vi "Variant to Datatype.vi"(4 "Variant":variant) -> (0 "Value":string, 1 "Name":string, 2 "Datatype":T1)   [LabVIEW 2019]
uses:
  Datatype.ctl
  <userlib>/_OpenG.lib/lvdata/lvdata.llb/Type Descriptor Enumeration__ogtk.ctl
  <vilib>/Utility/Data Type/NI_Data Type.lvlib
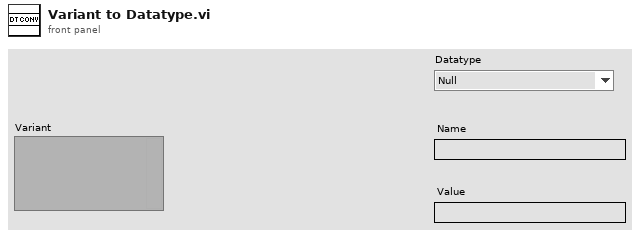
[diagram p1: front panel]
types:
  T1 = typedef "Datatype.ctl" = enum16{"Null", "Numeric", "String", "Bool", "Numeric 1D", "String 1D", "Bool 1D", "Numeric 2D", "String 2D", "Bool 2D", "Variant"}
  T2 = typedef "Type Descriptor Enumeration__ogtk.ctl" = enum8{"<Null>", "I8", "I16", "I32", "I64", "U8", "U16", "U32", "U64", "SGL", "DBL", "EXT", "CSG", "CDB", "CXT", "0x0F", "0x10", "0x11", "0x12", "0x13", "0x14", "Enum U8", "Enum U16", "Enum U32", "Enum U64", "SGL PQ", "DBL PQ", "EXT PQ", "CSG PQ", "CDB PQ", "CXT PQ", "0x1F", "0x20", "Boolean", "0x22", "0x23", "0x24", "0x25", "0x26", "0x27", "0x28", "0x29", "0x2A", "0x2B", "0x2C", "0x2D", "0x2E", "0x2F", "String", "0x31", "Path", "Pict", "0x34", "0x35", "0x36", "DAQ", "0x38", "0x39", "0x3A", "0x3B", "0x3C", "0x3D", "0x3E", "0x3F", "Array", "0x41", "0x42", "0x43", "0x44", "0x45", "0x46", "0x47", "0x48", "0x49", "0x4A", "0x4B", "0x4C", "0x4D", "0x4E", "0x4F", "Cluster", "0x51", "0x52", "Variant", "Waveform", "0x55", "0x56", "0x57", "0x58", "0x59", "0x5A", "0x5B", "0x5C", "0x5D", "0x5E", "Fixed Point", "0x60", "0x61", "0x62", "0x63", "0x64", "0x65", "0x66", "0x67", "0x68", "0x69", "0x6A", "0x6B", "0x6C", "0x6D", "0x6E", "0x6F", "Refnum", "0x71", "0x72", "Set Collection", "Map Collection"}
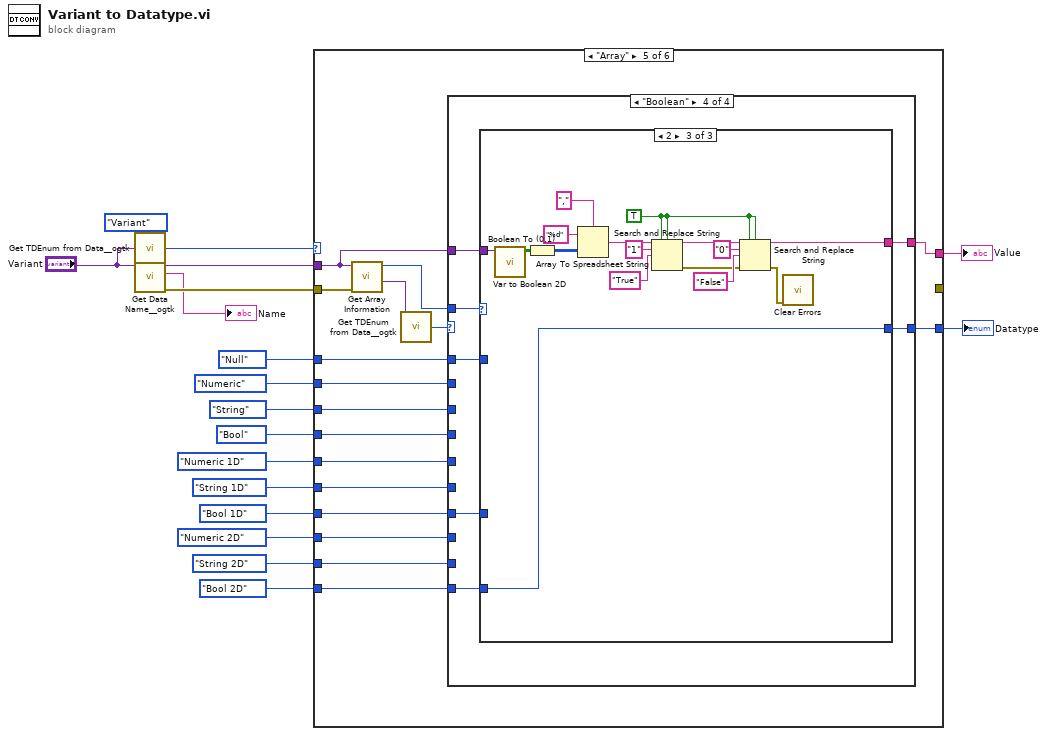
[diagram p0: block diagram]
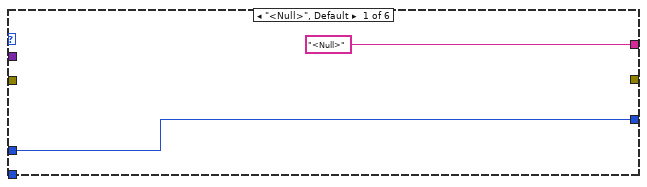
[diagram p2: hidden frame]
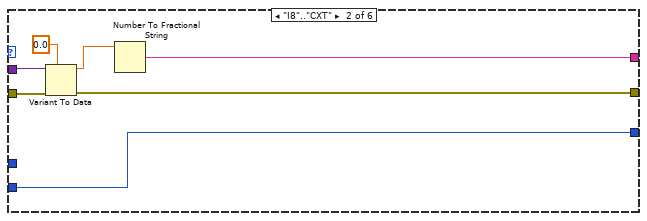
[diagram p3: hidden frame]
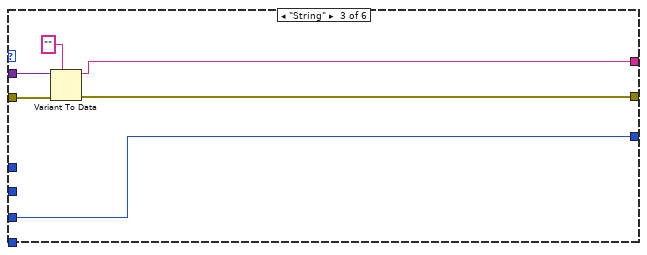
[diagram p4: hidden frame]
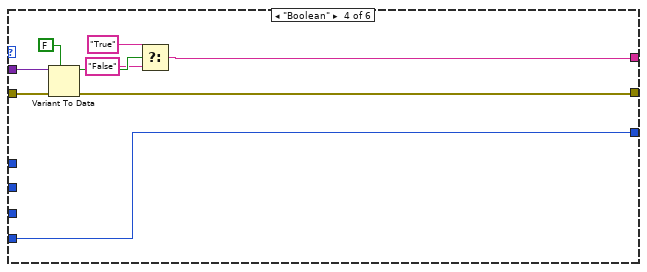
[diagram p5: hidden frame]
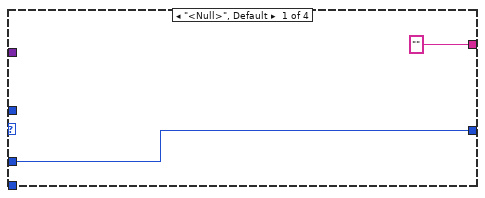
[diagram p6: hidden frame]
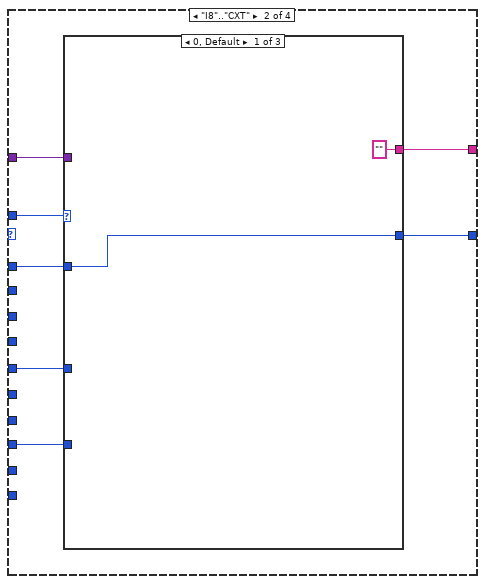
[diagram p7: hidden frame]
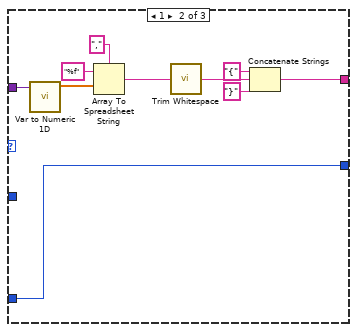
[diagram p8: hidden frame]
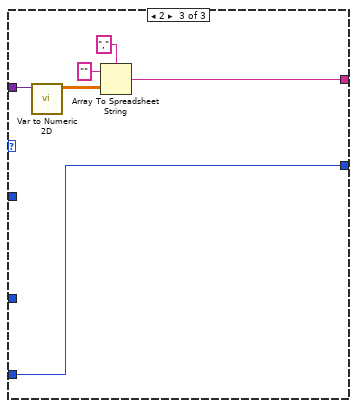
[diagram p9: hidden frame]
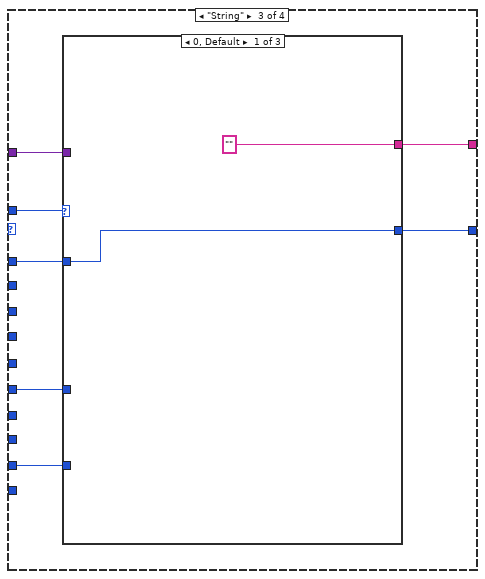
[diagram p10: hidden frame]
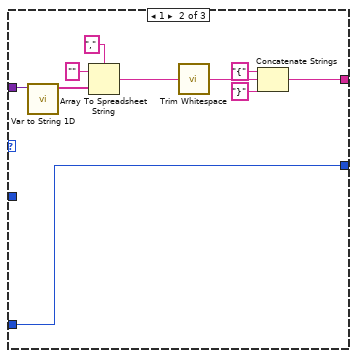
[diagram p11: hidden frame]
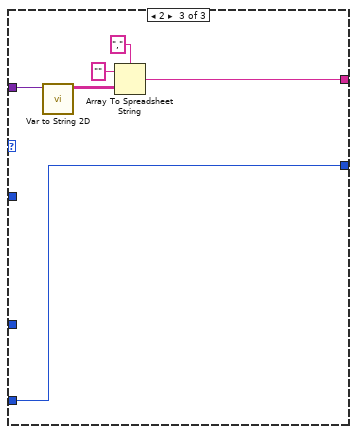
[diagram p12: hidden frame]
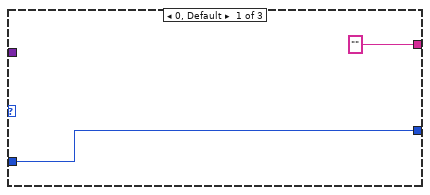
[diagram p13: hidden frame]
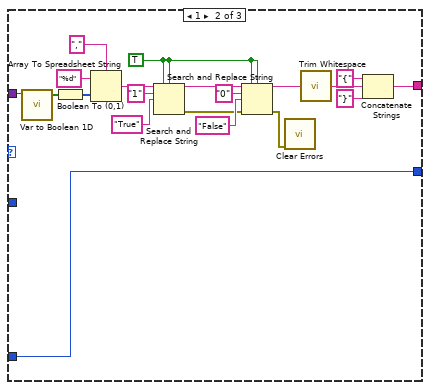
[diagram p14: hidden frame]
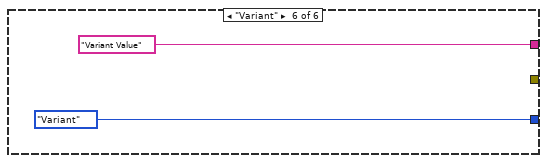
[diagram p15: hidden frame]
diagram:
  (unwired) Type_Descriptor_Enumeration__ogtk."Variant" ("Type Descriptor Enumeration")
  n1 = call <userlib>:"Get TDEnum from Data__ogtk.vi"("Data"="Variant") -> ("Type Descriptor Enumeration"=w11:T2)  [unwired: 4 in]
  n2 = call <userlib>:"Get Data Name__ogtk.vi"("Data"="Variant") -> ("error out"=w10:errorcluster, "Data Name"=→"Name":string, "Data dup"=w8:variant)  [unwired: 8 in]
  n3 = case shown="\"Array\"" w11 {
    tunnel: [w19 w26 w32 w41 w55 Datatype."Variant" ("Datatype")] -> w17
    tunnel: Datatype."Null" ("Datatype") -> [w19 _ _ _ w54 _]
    tunnel: Datatype."Numeric" ("Datatype") -> [_ w26 _ _ w53 _]
    tunnel: Datatype."String" ("Datatype") -> [_ _ w32 _ w52 _]
    tunnel: Datatype."Bool" ("Datatype") -> [_ _ _ w41 w51 _]
    tunnel: w10 -> [_ w24 w29 w38 w58 _]
    tunnel: w8 -> [_ w25 w30 w39 w43 _]
    tunnel: Datatype."Numeric 1D" ("Datatype") -> [_ _ _ _ w50 _]
    tunnel: Datatype."String 1D" ("Datatype") -> [_ _ _ _ w49 _]
    tunnel: Datatype."Bool 1D" ("Datatype") -> [_ _ _ _ w48 _]
    tunnel: Datatype."Numeric 2D" ("Datatype") -> [_ _ _ _ w47 _]
    tunnel: Datatype."String 2D" ("Datatype") -> [_ _ _ _ w46 _]
    tunnel: Datatype."Bool 2D" ("Datatype") -> [_ _ _ _ w45 _]
    tunnel: ["<Null>" w21 w28 w35 w42 "Variant Value"] -> w1
    tunnel: [_ w20 w27 w37 _ _] -> _
    frame "<Null>", Default {
    }
    frame "I8".."CXT" {
      n4 = Variant To Data(error in=w24, type=0.0, Variant=w25) -> (data=w22:dbl, error out=w20:errorcluster)
      n5 = Number To Fractional String(number=w22) -> (F-format string=w21:string)  [unwired: 3 in]
    }
    frame "String" {
      n6 = Variant To Data(error in=w29, type="", Variant=w30) -> (data=w28:string, error out=w27:errorcluster)
    }
    frame "Boolean" {
      n7 = Variant To Data(error in=w38, type=FALSE, Variant=w39) -> (data=w36:bool, error out=w37:errorcluster)
      n8 = Select(t="True", s=w36, f="False") -> (s? t:f=w35:string)
    }
    frame "Array" {
      n9 = call <vilib>:"Get Array Information.vi"("error in (no error)"=w58, "variant"=w43) -> ("array element data type"=w57:variant, "number of dimensions"=w44:i32)  [unwired: 6 in, 2 out]
      n10 = call <userlib>:"Get TDEnum from Data__ogtk.vi"("Data"=w57) -> ("Type Descriptor Enumeration"=w56:T2)  [unwired: 4 in]
      n11 = case shown="\"Boolean\"" w56 {
        tunnel: [w60 w61 w86 w116] -> w55
        tunnel: w54 -> [w60 w66 w92 w115]
        tunnel: w53 -> [_ _ _ _]
        tunnel: w52 -> [_ _ _ _]
        tunnel: w51 -> [_ _ _ _]
        tunnel: w50 -> [_ w65 _ _]
        tunnel: w49 -> [_ _ w90 _]
        tunnel: w48 -> [_ _ _ w114]
        tunnel: w47 -> [_ w64 _ _]
        tunnel: w46 -> [_ _ w89 _]
        tunnel: w45 -> [_ _ _ w113]
        tunnel: w44 -> [_ w67 w91 w117]
        tunnel: w43 -> [_ w63 w88 w112]
        tunnel: ["" ("spreadsheet string") w62 w87 w111] -> w42
        frame "<Null>", Default {
        }
        frame "I8".."CXT" {
          n12 = case shown="0, Default" w67 {
            tunnel: [w69 w79 w85] -> w61
            tunnel: w66 -> [w69 _ _]
            tunnel: w65 -> [_ w79 _]
            tunnel: w64 -> [_ _ w85]
            tunnel: w63 -> [_ w76 w81]
            tunnel: ["" w72 w82] -> w62
            frame 0, Default {
            }
            frame 1 {
              n13 = call "Var to Numeric 1D.vi"("Variant"=w76) -> ("Numeric Array"=w75:dbl[])  [unwired: 10 in]
              n14 = Array To Spreadsheet String(delimiter (Tab)=",", array=w75, 3:"%f" ("format string")) -> (spreadsheet string=w74:string)
              n15 = call <vilib>:"Trim Whitespace.vi"("string"=w74) -> ("trimmed string"=w73:string)  [unwired: 1 in]
              n16 = Concatenate Strings("{" ("string"), w73, "}" ("string")) -> (w72:string)
            }
            frame 2 {
              n17 = call "Var to Numeric 2D.vi"("Variant"=w81) -> ("Numeric Array"=w80:dbl[][])  [unwired: 10 in]
              n18 = Array To Spreadsheet String(delimiter (Tab)=",", array=w80, 3:"" ("format string")) -> (spreadsheet string=w82:string)
            }
          }
        }
        frame "String" {
          n19 = case shown="0, Default" w91 {
            tunnel: [w94 w104 w110] -> w86
            tunnel: w92 -> [w94 _ _]
            tunnel: w90 -> [_ w104 _]
            tunnel: w89 -> [_ _ w110]
            tunnel: w88 -> [_ w103 w107]
            tunnel: ["" ("spreadsheet string") w95 w105] -> w87
            frame 0, Default {
            }
            frame 1 {
              n20 = call "Var to String 1D.vi"("Variant"=w103) -> ("String 1D"=w102:string[])  [unwired: 10 in]
              n21 = Array To Spreadsheet String(delimiter (Tab)=",", array=w102, 3:"" ("format string")) -> (spreadsheet string=w96:string)
              n22 = call <vilib>:"Trim Whitespace.vi"("string"=w96) -> ("trimmed string"=w99:string)  [unwired: 1 in]
              n23 = Concatenate Strings("{" ("string"), w99, "}" ("string")) -> (w95:string)
            }
            frame 2 {
              n24 = call "Var to String 2D.vi"("Variant"=w107) -> ("String 2D"=w106:string[][])  [unwired: 10 in]
              n25 = Array To Spreadsheet String(delimiter (Tab)=",", array=w106, 3:"" ("format string")) -> (spreadsheet string=w105:string)
            }
          }
        }
        frame "Boolean" {
          n26 = case shown="2" w117 {
            tunnel: [w119 w139 w155] -> w116
            tunnel: w115 -> [w119 _ _]
            tunnel: w114 -> [_ w139 _]
            tunnel: w113 -> [_ _ w155]
            tunnel: w112 -> [_ w128 w141]
            tunnel: ["" w120 w142] -> w111
            frame 0, Default {
            }
            frame 1 {
              w129 = TRUE ("replace all? (F)")
              n27 = call "Var to Boolean 1D.vi"("Variant"=w128) -> ("Bool 1D"=w127:bool[])  [unwired: 10 in]
              n28 = Boolean To (0,1)(Boolean=w127) -> (0, 1=w138:i16[])
              n29 = Array To Spreadsheet String(delimiter (Tab)=",", array=w138, 3:"%d" ("format string")) -> (spreadsheet string=w135:string)
              n30 = Search and Replace String(replace all?=w129, case sensitive?=w129, input string=w135, search string="1", replace string="True" ("replace string (\"\")")) -> (result string=w132:string, error out=w126:errorcluster)  [unwired: 3 in, 2 out]
              n31 = Search and Replace String(replace all?=w129, case sensitive?=w129, input string=w132, search string="0", replace string="False" ("replace string (\"\")"), error in=w126) -> (result string=w121:string, error out=w125:errorcluster)  [unwired: 2 in, 2 out]
              n32 = call <vilib>:"Clear Errors.vi"("error in (no error)"=w125) -> ()  [unwired: 5 in, 2 out]
              n33 = call <vilib>:"Trim Whitespace.vi"("string"=w121) -> ("trimmed string"=w124:string)  [unwired: 1 in]
              n34 = Concatenate Strings("{" ("string"), w124, "}" ("string")) -> (w120:string)
            }
            frame 2 {
              w145 = TRUE ("replace all? (F)")
              n35 = call "Var to Boolean 2D.vi"("Variant"=w141) -> ("Bool 2D"=w140:bool[][])  [unwired: 10 in]
              n36 = Boolean To (0,1)(Boolean=w140) -> (0, 1=w154:i16[][])
              n37 = Array To Spreadsheet String(delimiter (Tab)=",", array=w154, 3:"%d" ("format string")) -> (spreadsheet string=w151:string)
              n38 = Search and Replace String(replace all?=w145, case sensitive?=w145, input string=w151, search string="1", replace string="True" ("replace string (\"\")")) -> (result string=w148:string, error out=w144:errorcluster)  [unwired: 3 in, 2 out]
              n39 = Search and Replace String(replace all?=w145, case sensitive?=w145, input string=w148, search string="0", replace string="False" ("replace string (\"\")"), error in=w144) -> (result string=w142:string, error out=w143:errorcluster)  [unwired: 2 in, 2 out]
              n40 = call <vilib>:"Clear Errors.vi"("error in (no error)"=w143) -> ()  [unwired: 5 in, 2 out]
            }
          }
        }
      }
    }
    frame "Variant" {
    }
  }
  "Datatype" <- w17
  "Value" <- w1
